vi "TemplateGUITAF_SendUiEvent.vi"(7 "UiEventNames":T1, 8 "ErrorIn":errorcluster, 9 "Data":variant, 11 "TemplateGUITAFIn":refnum<class "TemplateGUITAF.lvclass">) -> (0 "ErrorOut":errorcluster, 3 "TemplateGUITAFOut":refnum<class "TemplateGUITAF.lvclass">)   [LabVIEW 2021, in "TemplateGUITAF.lvlib" / "TemplateGUITAF.lvclass"]
doc: "Sends the selected event to the registered event handler loops in the user interface VI."
uses:
  TemplateGUITAF.lvclass
  TemplateGUITAF_UiCallBackEvents.ctl
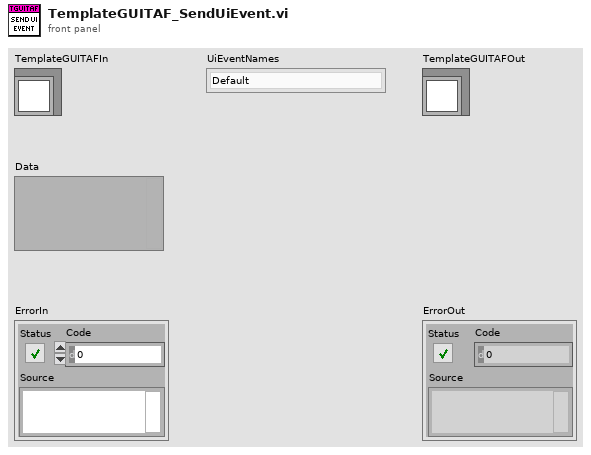
[diagram p1: front panel]
types:
  T1 = typedef "TemplateGUITAF.lvlib/TemplateGUITAF.lvclass/TemplateGUITAF_UiCallBackEvents.ctl" = enum16{"Default", "PersistentDataUpdated"}
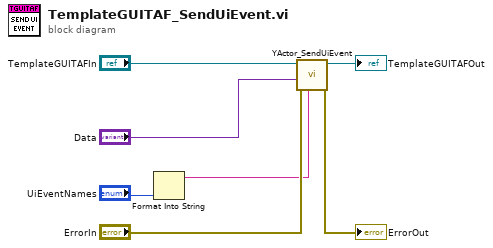
[diagram p0: block diagram]
diagram:
  n1 = Format Into String("UiEventNames") -> (resulting string=w2:string)  [unwired: 3 in, 1 out]
  n2 = call-dynamic "YActor_SendUiEvent.vi"("Event"=w2, "ErrorIn"="ErrorIn", "Data"="Data", "YActorIn"="TemplateGUITAFIn") -> ("ErrorOut"=→"ErrorOut":errorcluster, "YActorOut"=→"TemplateGUITAFOut":refnum<class "TemplateGUITAF.lvclass">)  [unwired: 6 in]
